vi "Table to JSON Schema.vi"(8 "error in (no error)":errorcluster, 10 "Table":string[][](table), 11 "JSON Schema in":string) -> (0 "error out":errorcluster, 3 "JSON Schema out":string)   [LabVIEW 2019, in "JSON-Schema.lvlib"]
doc: "<b>InfoTable</b> is a table.\n- First row: name, description, units, (min_value, min_value)\n- Remainder: values"
uses:
  JSON-Schema.lvlib
  92616eff-9b0c-4e28-944c-aab5ae23ad69.vi
  <vilib>/JDP Science/JSONtext/Next JSON Value.vi
  <vilib>/JDP Science/JSONtext/String Subset.vi
  <vilib>/JDP Science/JSONtext/Parsing/Advance past next JSON Value (inlined COPY).vi
  <vilib>/JDP Science/JSONtext/Parsing/Advance past whitespace.vi
  <vilib>/JDP Science/JSONtext/Parsing/Advance past String.vi
  <vilib>/JDP Science/JSONtext/Parsing/Advance past Number.vi
  <vilib>/JDP Science/JSONtext/Parsing/Advance past Line Ending.vi
  <vilib>/JDP Science/JSONtext/Parsing/Parse Full Path or Item Name.vi
  <vilib>/JDP Science/JSONtext/Parsing/Advance past Array.vi
  <vilib>/JDP Science/JSONtext/Parsing/Advance past Object.vi
  <vilib>/JDP Science/JSONtext/support/Error Cluster From Code.vi
  <vilib>/JDP Science/JSONtext/Offset/Find Item Locations by Path.vi
  <vilib>/JDP Science/JSONtext/Variant to JSON Text.vi
  <vilib>/JDP Science/JSONtext/LVClass Serializer/JSONtext LVClass Serializer.lvclass
  <vilib>/JDP Science/JSONtext/JSONtext.lvlib
panel:
  in  "Object Name":string
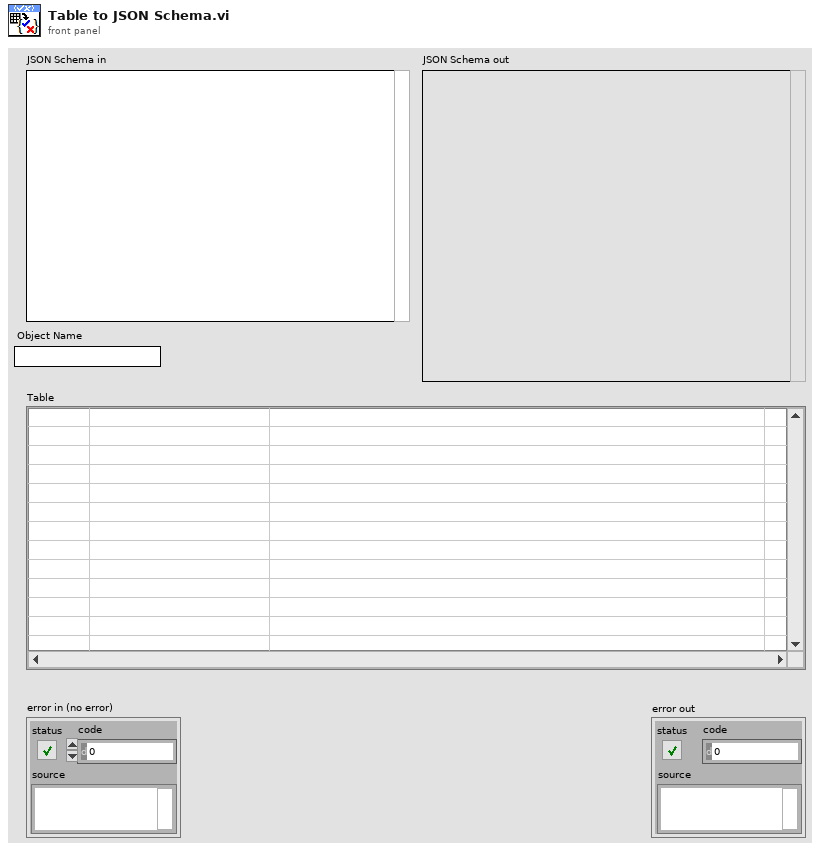
[diagram p1: front panel]
types:
  T1 = typedef "JSONtext.lvlib/JSON Value Type.ctl" = enum16{"Not a JSON Value", "JSON Object", "JSON Array", "String", "Number", "true", "false", "null"}
  T2 = enum32{"Bad", "Idle", "Run top level", "Running"}
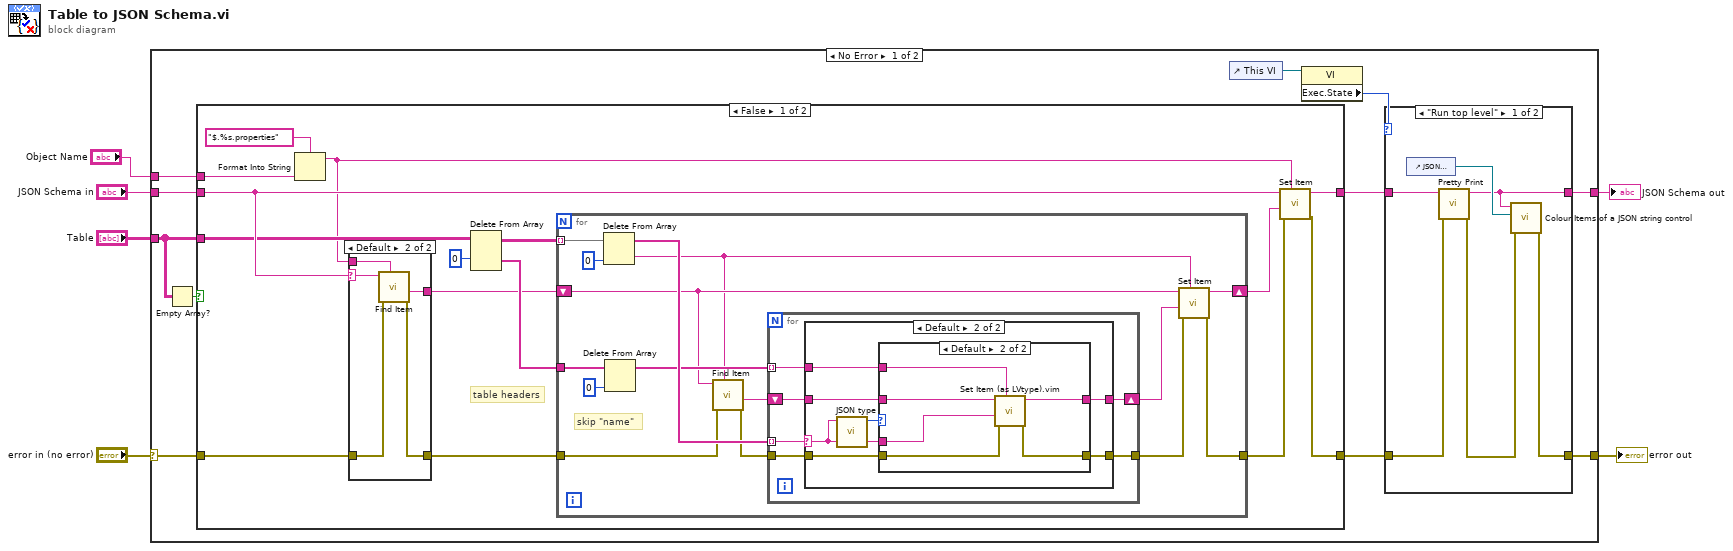
[diagram p0: block diagram]
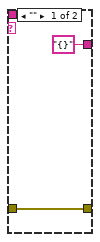
[diagram p2: hidden frame]
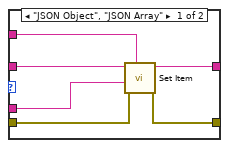
[diagram p4: hidden frame]
diagram:
  n1 = case shown="No Error" "error in (no error)" {
    selector: "error in (no error)" -> [w17 w92]
    tunnel: "Table" -> [w9 _]
    tunnel: [w12 w92] -> w5
    tunnel: "JSON Schema in" -> [w16 _]
    tunnel: [w11 _] -> w3
    tunnel: "Object Name" -> [w7 _]
    frame No Error {
      n2 = Empty Array?(array=w9) -> (empty?=w8:bool)
      n3 = case shown="False" w8 {
        tunnel: w17 -> [w28 w82]
        tunnel: w16 -> [w24 w83]
        tunnel: [w23 w83] -> w13
        tunnel: [w22 w82] -> w10
        tunnel: w9 -> [w21 _]
        tunnel: w7 -> [w18 _]
        frame False {
          # "table headers"
          n4 = Format Into String(format string="$.%s.properties" ("$Path or Item Name"), w18) -> (resulting string=w19:string)  [unwired: 2 in, 1 out]
          n5 = case shown="Default" w24 {
            selector: w24 -> [_ w36]
            tunnel: ["{}" ("<JSON>") w39] -> w29
            tunnel: w28 -> [w33 w38]
            tunnel: [w33 w37] -> w27
            tunnel: w19 -> [_ w35]
            frame "" {
            }
            frame Default {
              n6 = call <vilib>:"Find Item.vi"("$Path or Item Name"=w35, "error in (no error)"=w38, "JSON"=w36) -> ("error out"=w37:errorcluster, "<JSON>"=w39:string)  [unwired: 5 in, 2 out]
            }
          }
          n7 = Delete From Array(array=w21, index (row)=0) -> (deleted portion=w30:string[], array with subset deleted=w32:string[][])  [unwired: 2 in]
          n8 = for {
            tunnel: w32 -> [w54] mode=indexing
            shift-right: [w51] -> w26
            shift-left: w29 -> [w44]
            tunnel: w30 -> [w48]
            tunnel: [w49] -> w25
            tunnel: w27 -> [w40]
            # "skip \"name\""
            n9 = Delete From Array(array=w54, index=0) -> (deleted portion=w43:string, array with subset deleted=w53:string[])  [unwired: 1 in]
            n10 = Delete From Array(array=w48, index=0) -> (array with subset deleted=w45:string[])  [unwired: 1 in, 1 out]
            n11 = call <vilib>:"Find Item.vi"("$Path or Item Name"=w43, "error in (no error)"=w40, "JSON"=w44) -> ("error out"=w41:errorcluster, "<JSON>"=w42:string)  [unwired: 5 in, 2 out]
            n12 = for {
              tunnel: w53 -> [w55] mode=indexing
              tunnel: w45 -> [w56] mode=indexing
              shift-right: [w59] -> w52
              shift-left: w42 -> [w60]
              tunnel: [w58] -> w50
              tunnel: w41 -> [w57]
              n13 = case shown="Default" w55 {
                selector: w55 -> [_ w63]
                tunnel: w60 -> [w62 w69]
                tunnel: [w62 w68] -> w59
                tunnel: [w61 w67] -> w58
                tunnel: w57 -> [w61 w66]
                tunnel: w56 -> [_ w65]
                frame "" {
                }
                frame Default {
                  n14 = call <vilib>:"JSON type.vi"("JSON"=w63) -> ("JSON Value Type"=w64:T1)  [unwired: 9 in, 1 out]
                  n15 = case shown="Default" w64 {
                    tunnel: w69 -> [w75 w78]
                    tunnel: [w74 w79] -> w68
                    tunnel: [w70 w76] -> w67
                    tunnel: w66 -> [w71 w77]
                    tunnel: w65 -> [w73 w81]
                    tunnel: w63 -> [w72 w80]
                    frame "JSON Object", "JSON Array" {
                      n16 = call <vilib>:"Set Item.vi"("$Path or Item Name"=w73, "error in (no error)"=w71, "JSON to Insert"=w72, "JSON"=w75) -> ("error out"=w70:errorcluster, "<JSON>"=w74:string)  [unwired: 4 in, 1 out]
                    }
                    frame Default {
                      n17 = call "Set Item (as LVtype).vim"("$Path or Item Name"=w81, "error in (no error)"=w77, "Anything"=w80, "JSON"=w78) -> ("error out"=w76:errorcluster, "<JSON>"=w79:string)  [unwired: 4 in, 1 out]
                    }
                  }
                }
              }
            }
            n18 = call <vilib>:"Set Item.vi"("$Path or Item Name"=w43, "error in (no error)"=w50, "JSON to Insert"=w52, "JSON"=w44) -> ("error out"=w49:errorcluster, "<JSON>"=w51:string)  [unwired: 4 in, 1 out]
          }
          n19 = call <vilib>:"Set Item.vi"("$Path or Item Name"=w19, "error in (no error)"=w25, "JSON to Insert"=w26, "JSON"=w24) -> ("error out"=w22:errorcluster, "<JSON>"=w23:string)  [unwired: 4 in, 1 out]
        }
        frame True {
        }
      }
      n20 = control-ref of="This VI"() -> (w15:refnum<vi>)
      n21 = property class="VI"(reference=w15) -> ("Exec.State"=w14:T2)  [unwired: 1 in, 2 out]
      n22 = case shown="\"Run top level\"" w14 {
        tunnel: w10 -> [w88 w90]
        tunnel: w13 -> [w87 w91]
        tunnel: [w86 w90] -> w12
        tunnel: [w84 w91] -> w11
        frame "Run top level" {
          n23 = control-ref of="JSON Schema out"() -> (w89:refnum<vi>)
          n24 = call <vilib>:"Pretty Print.vi"("error in (no error)"=w88, "JSON"=w87) -> ("error out"=w85:errorcluster, "<JSON>"=w84:string)  [unwired: 7 in, 1 out]
          n25 = call <vilib>:"Colour Items of a JSON string control.vi"("error in (no error)"=w85, "String Control"=w89, "JSON"=w84) -> ("error out"=w86:errorcluster)  [unwired: 8 in]
        }
        frame Default {
        }
      }
    }
    frame Error {
    }
  }
  "JSON Schema out" <- w3
  "error out" <- w5
